vi "VALEW_ATC_Verify Non-concurrent.vi"(0 "GEA2 Reference In":refnum<k24>, 11 "Error In":errorcluster) -> (4 "GEA2 Reference Out":refnum<k24>, 6 "Pass/fail?":bool, 8 "Report Text":string, 15 "Error Out":errorcluster)   [LabVIEW 2016, in "TL27.lvlib"]
doc: "This test covers the ATC algorithm when doing a non-concurrent fill. A non-concurrent fill does not allow both hot and cold valves to be on at the same time. The valves are operated in series, not in parallel."
uses:
  Projects/TL27.lvlib
  C:/Automation/DLLs/PC Dot Net/GeaCommunication.dll
  Common/LabVIEW GEA2 Toolkit/LabVIEW_GEA2_Toolkit.lvlibp/type defs/Source_Destination.ctl
  Valew Common/type defs/MC_Cycle_Engine_Request_State.ctl
  Common/LabVIEW GEA2 Toolkit/LabVIEW_GEA2_Toolkit.lvlibp/type defs/ERD Write Data In.ctl
  Common/LabVIEW GEA2 Toolkit/LabVIEW_GEA2_Toolkit.lvlibp/type defs/Data Type.ctl
  Common/LabVIEW GEA2 Toolkit/LabVIEW_GEA2_Toolkit.lvlibp/type defs/ERD Read Data In.ctl
  <vilib>/DAQmx/write.llb/DAQmx Write (Analog DBL 1Chan 1Samp).vi
  <vilib>/DAQmx/create/channels.llb/DAQmx Create Channel (AO-Voltage-Basic).vi
  <vilib>/DAQmx/miscellaneous.llb/DAQmx Fill In Error Info.vi
  Common/LabVIEW GEA2 Toolkit/LabVIEW_GEA2_Toolkit.lvlibp
panel:
  out "Hot valve time (s) ATC 2":u16
  out "Cold valve time (s) ATC 2":u16
  out "Cold valve time (s) Calc 2":dbl
  out "Hot valve time (s) Calc 2":dbl
  out "High Times (s)":dbl[][](array[numeric])=[[0.048, 19.932000000000002, 0.0], [0.256, 9.626, 10.098], [0.254, 9.628, 10.098], [0.256, 9.625, 10.099], [0.047, 19.933, 0.0], [0.253, 10.701, 9.026], [0.255, 10.699, 9.026], [0.048, 19.932000000000002, 0.0], [0.258, 8.014, 11.708], [0.256, 8.016, 11.708], [0.256, 8.016, 11.708], [0.048, 19.932000000000002, 0.0], [0.254, 7.527, 12.199], [0.047, 19.933, 0.0], [0.253, 6.848, 12.879]]
  out "Hot inlet temp updated after 30sec?":bool
  out "Calc bath temp after seg gals":dbl
  out "Bath temp after seg gals":dbl
  out "Hot valve time (s) ATC":u16
  out "Cold valve time (s) ATC":u16
  out "Bath temp updated after segment fill?":bool
  out "Cold inlet temp updated after 30sec?":bool
  out "Cold valve pass?":bool
  out "Hot valve pass?":bool
  out "Cold valve time (s) Calc":dbl
  out "Hot valve time (s) Calc":dbl
  in  "Standalone?":bool
  # "Segment 1"
  # "Segment 2"
  # "off"
  # "on"
  # "off"
  # "on"
  # "off"
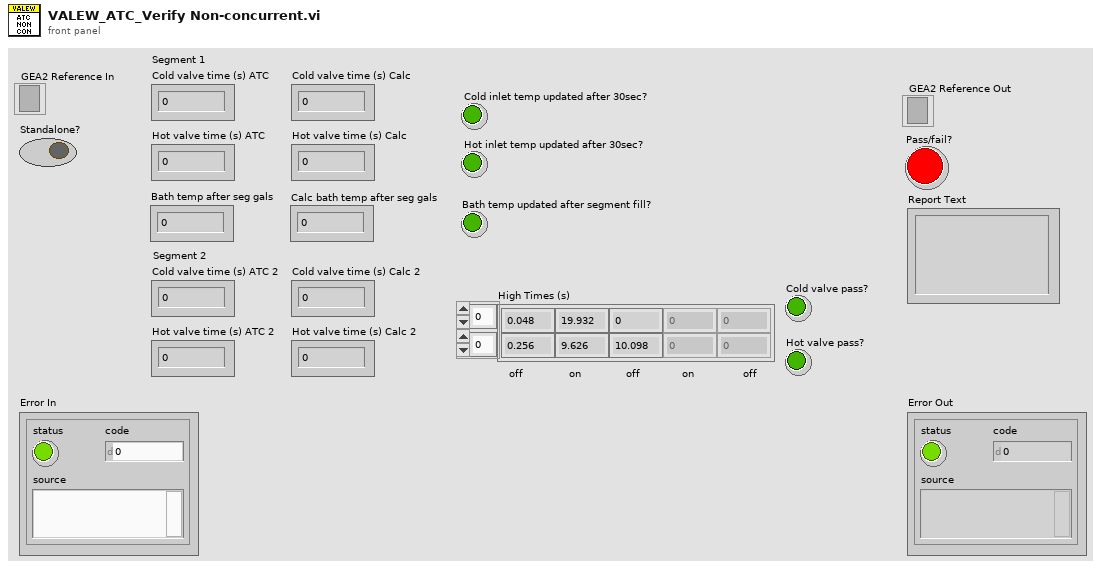
[diagram p1: front panel]
types:
  T1 = typedef "LabVIEW_GEA2_Toolkit.lvlibp/ERD Write Data In.ctl" = cluster{"ERD Number":u16, "Data Type":T2, "Data":string}
  T2 = typedef "LabVIEW_GEA2_Toolkit.lvlibp/Data Type.ctl" = enum16{"string", "boolean", "uint8_t", "uint16_t", "uint32_t", "uint64_t", "int8_t", "int16_t", "int32_t", "int64_t"}
  T3 = typedef "LabVIEW_GEA2_Toolkit.lvlibp/ERD Read Data In.ctl" = cluster{"ERD Number":u16, "Data Type":T2}
  T4 = enum16{"EQ (==)", "NE (!=)", "GT (>)", "LT (<)", "GE (>=)", "LE (<=)", "GTLT(> <)", "GELE (>= <=)", "GELT (>= <)", "GTLE (> <=)", "LTGT (< >)", "LEGE (<= >=)", "LEGT (<= >)", "LTGE (< >=)", "No Comparison"}
  T5 = typedef "TL27.lvlib/MC_Cycle_Engine_Request_State.ctl" = enum16{"Select", "Start", "Pause", "Resume", "Stop"}
  T6 = typedef "LabVIEW_GEA2_Toolkit.lvlibp/Source_Destination.ctl" = cluster{"Source":u8, "Destination":u8}
  T7 = typedef "TL27.lvlib/VALEW_ATC_Data.ctl" = cluster{"Accumulated hot gallons":dbl, "Accumulated cold gallons":dbl, "Current tub gallons":dbl, "Cold inlet temp (F)":dbl, "Hot inlet temp (F)":dbl, "Warm inlet temp (F)":dbl, "Hot valve time (s)":u16, "Cold valve time (s)":u16, "Current bath temp (F)":dbl, "Current water temp (F)":dbl, "Segment gallons":dbl}
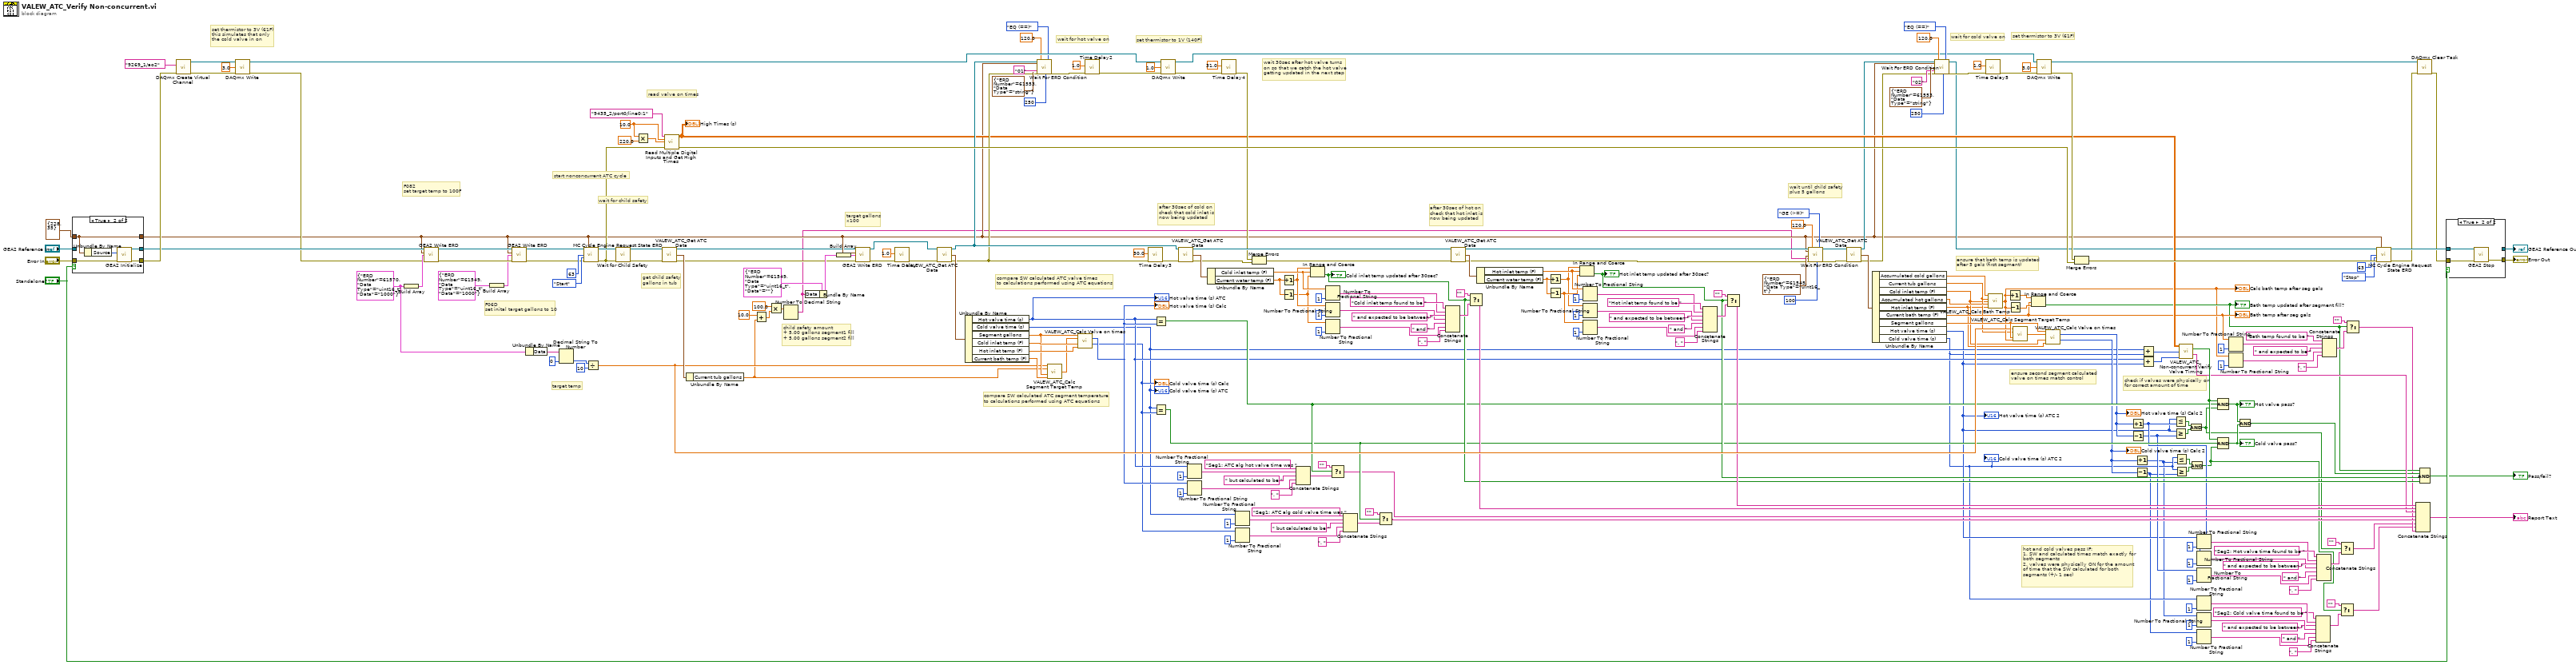
[diagram p0: block diagram]
diagram:
  w199 = 10.0 ("rate")
  w236 = T1 {"ERD Number"=61570, "Data Type"=enum."uint16_t", "Data"="1000"} ("ERD Write Data In")
  # "wait until child safety\nplus 5 gallons"
  # "hot and cold valves pass IF:\n1. SW and calculated times match exactly for\nboth segments\n2. valves were physically ON for the amount\nof time that the SW calculated for both\nsegments (+/- 1 sec)"
  # "compare SW calculated ATC valve times\nto calculations performed using ATC equations"
  # "compare SW calculated ATC segment temperature\nto calculations performed using ATC equations"
  # "wait 30sec after hot valve turns\non so that we catch the hot valve\ngetting updated in the next step"
  # "F06D\nset inital target gallons to 10"
  # "target gallons\nx100"
  # "check if valves were physically on\nfor correct amount of time"
  # "ensure second segment calculated\nvalve on times match control"
  # "ensure that bath temp is updated\nafter 5 gals (first segment)"
  # "wait for cold valve on"
  # "set thermistor to 3V (61F)"
  # "wait for hot valve on"
  # "set thermistor to 1V (140F)"
  # "after 30sec of hot on\ncheck that hot inlet is\nnow being updated"
  # "child safety amount\n+ 5.00 gallons segment1 fill\n+ 5.00 gallons segment2 fill"
  # "after 30sec of cold on\ncheck that cold inlet is\nnow being updated"
  # "get child safety\ngallons in tub"
  # "read valve on times"
  # "target temp"
  # "set thermistor to 3V (61F)\nthis simulates that only\nthe cold valve in on"
  # "wait for child safety"
  # "start nonconcurrent ATC cycle"
  # "F082\nset target temp to 100F"
  n1 = case shown="True" "Standalone?" {
    tunnel: T6 {"Source"=228, "Destination"=35} ("GEA Inputs") -> [w247 w250]
    tunnel: [w249 w253] -> w149
    tunnel: [w248 w252] -> w211
    tunnel: "Error In" -> [w248 w251]
    tunnel: "GEA2 Reference In" -> [w249 _]
    tunnel: [w247 w250] -> w7
    frame False {
    }
    frame True {
      n2 = Unbundle By Name(w250) -> ("Source"=w254:u8)
      n3 = call "GEA2 Initialize.vi"("Source Address"=w254, "error in"=w251) -> ("GEA2 Reference Out"=w253:refnum<k24>, "error out"=w252:errorcluster)  [unwired: 11 in, 1 out]
    }
  }
  n4 = call-poly <vilib>:"DAQmx Create Virtual Channel.vi"("physical channels"=tag "9269_1/ao2", "error in"=w211) -> ("task out"=w228:refnum<k21>, "error out"=w227:errorcluster)  [unwired: 12 in]
  n5 = call-poly <vilib>:"DAQmx Write.vi"("task/channels in"=w228, "data"=3.0, "error in"=w227) -> ("task out"=w196:refnum<k21>, "error out"=w148:errorcluster)  [unwired: 10 in, 1 out]
  n6 = Build Array(w236) -> (w235:T1[])
  n7 = call "GEA2 Write ERD.vi"("GEA2 Reference In"=w149, "GEA Inputs"=w7, "Write ERD List"=w235, "Error In"=w148) -> ("GEA2 Reference Out"=w224:refnum<k24>, "Error Out"=w223:errorcluster)  [unwired: 9 in, 1 out]
  n8 = Build Array(T1 {"ERD Number"=61549, "Data Type"=enum."uint16_t", "Data"="1000"} ("ERD Write Data In")) -> (w207:T1[])
  n9 = call "GEA2 Write ERD.vi"("GEA2 Reference In"=w224, "GEA Inputs"=w7, "Write ERD List"=w207, "Error In"=w223) -> ("GEA2 Reference Out"=w221:refnum<k24>, "Error Out"=w222:errorcluster)  [unwired: 9 in, 1 out]
  n10 = Unbundle By Name(w236) -> ("Data"=w234:string)
  n11 = Decimal String To Number(string=w234, default (0L)=u16 0 ("default (0 U32)")) -> (number=w232:u16)  [unwired: 1 in, 1 out]
  n12 = call "MC Cycle Engine Request State ERD.vi"("GEA2 Reference In"=w221, "GEA Inputs"=w7, "Cycle #"=u8 63, "MC Cycle Engine State"=MC_Cycle_Engine_Request_State."Start", "Error In"=w222) -> ("GEA2 Reference Out"=w241:refnum<k24>, "Error Out"=w160:errorcluster)  [unwired: 9 in]
  n13 = Divide(x=w232, y=u16 10) -> (x/y=w154:dbl)
  n14 = call "Wait for Child Safety.vi"("GEA2 Reference In"=w241, "Error In"=w160) -> ("GEA2 Reference Out"=w220:refnum<k24>, "Error Out"=w195:errorcluster)  [unwired: 9 in, 3 out]
  n15 = Multiply(x=w199, y=220.0) -> (x*y=w200:dbl)
  n16 = call "VALEW_ATC_Get ATC Data.vi"("GEA2 Reference In"=w220, "Error In"=w195) -> ("GEA2 Reference Out"=w2:refnum<k24>, "ATC Data"=w219:T7, "Error Out"=w5:errorcluster)  [unwired: 11 in]
  n17 = call "Read Multiple Digital Inputs and Get High Times.vi"("Lines"=tag "9435_2/port0/line0:1", "Rate (Hz)"=w199, "Samples"=w200, "Error In"=w160) -> ("High Times (s)"=w159:dbl[][], "Error Out"=w198:errorcluster)  [unwired: 10 in]
  "High Times (s)" <- w159
  n18 = Unbundle By Name(w219) -> ("Current tub gallons"=w6:dbl)
  n19 = Add(x=10.0, y=w6) -> (x+y=w9:dbl)
  n20 = Multiply(x=100.0, y=w9) -> (x*y=w10:dbl)
  n21 = Number To Decimal String(number=w10) -> (decimal integer string=w1:string)  [unwired: 1 in]
  n22 = Bundle By Name(cluster=T1 {"ERD Number"=61549, "Data Type"=enum."uint16_t", "Data"=""} ("ERD Write Data In"), "Data"=w1) -> (w11:T1)
  n23 = Build Array(w11) -> (w14:T1[])
  n24 = call "GEA2 Write ERD.vi"("GEA2 Reference In"=w2, "GEA Inputs"=w7, "Write ERD List"=w14, "Error In"=w5) -> ("GEA2 Reference Out"=w3:refnum<k24>, "Error Out"=w4:errorcluster)  [unwired: 9 in, 1 out]
  n25 = call "Time Delay"("error in (no error)"=w4, "Delay Time (s)"=1.0) -> ("error out"=w239:errorcluster)  [unwired: 9 in]
  n26 = call "VALEW_ATC_Get ATC Data.vi"("GEA2 Reference In"=w3, "Error In"=w239) -> ("GEA2 Reference Out"=w178:refnum<k24>, "ATC Data"=w238:T7, "Error Out"=w170:errorcluster)  [unwired: 11 in]
  n27 = Unbundle By Name(w238) -> ("Hot valve time (s)"=w29:u16, "Cold valve time (s)"=w27:u16, "Segment gallons"=w209:dbl, "Cold inlet temp (F)"=w217:dbl, "Hot inlet temp (F)"=w237:dbl, "Current bath temp (F)"=w208:dbl)
  "Cold valve time (s) ATC" <- w27
  "Hot valve time (s) ATC" <- w29
  n28 = call "Wait For ERD Condition.vi"("GEA2 Reference In"=w178, "GEA Inputs"=w7, "ERD Read Data"=T3 {"ERD Number"=61553, "Data Type"=enum."string"}, "Expected Low"="01", "Error In"=w170, "Timeout (s)"=120.0, "Loop Rate (ms)"=u32 250, "Comparison"=T4."EQ (==)") -> ("Error Out"=w167:errorcluster)  [unwired: 7 in, 4 out]
  n29 = call "VALEW_ATC_Calc Segment Target Temp.vi"("T(target)"=w154, "V(bath)"=w6, "V(segment)"=w209, "T(bath)"=w208) -> ("T(segment target)"=w210:dbl)  [unwired: 11 in]
  n30 = call "VALEW_ATC_Calc Valve on times.vi"("V(segment)"=w209, "T(segment target)"=w210, "T(cold inlet)"=w217, "T(hot inlet)"=w237) -> ("t(hot valve)"=w30:u16, "t(cold valve)"=w28:u16)  [unwired: 10 in]
  "Hot valve time (s) Calc" <- w30
  "Cold valve time (s) Calc" <- w28
  n31 = call "Time Delay2"("error in (no error)"=w167, "Delay Time (s)"=1.0) -> ("error out"=w168:errorcluster)  [unwired: 9 in]
  n32 = call "Time Delay3"("error in (no error)"=w170, "Delay Time (s)"=30.0) -> ("error out"=w193:errorcluster)  [unwired: 9 in]
  n33 = Equal?(x=w29, y=w30) -> (x = y?=w75:bool)
  n34 = Equal?(x=w27, y=w28) -> (x = y?=w74:bool)
  n35 = call-poly <vilib>:"DAQmx Write.vi"("task/channels in"=w196, "data"=1.0, "error in"=w168) -> ("task out"=w171:refnum<k21>, "error out"=w191:errorcluster)  [unwired: 10 in, 1 out]
  n36 = call "VALEW_ATC_Get ATC Data.vi"("GEA2 Reference In"=w178, "Error In"=w193) -> ("GEA2 Reference Out"=w188:refnum<k24>, "ATC Data"=w229:T7, "Error Out"=w185:errorcluster)  [unwired: 11 in]
  n37 = Number To Fractional String(number=w29, precision (6)=i16 1) -> (F-format string=w91:string)  [unwired: 2 in]
  n38 = Number To Fractional String(number=w30, precision (6)=i16 1) -> (F-format string=w89:string)  [unwired: 2 in]
  n39 = Unbundle By Name(w229) -> ("Cold inlet temp (F)"=w110:dbl, "Current water temp (F)"=w216:dbl)
  n40 = call "Time Delay4"("error in (no error)"=w191, "Delay Time (s)"=31.0) -> ("error out"=w163:errorcluster)  [unwired: 9 in]
  n41 = Number To Fractional String(number=w27, precision (6)=i16 1) -> (F-format string=w78:string)  [unwired: 2 in]
  n42 = Number To Fractional String(number=w28, precision (6)=i16 1) -> (F-format string=w80:string)  [unwired: 2 in]
  n43 = Merge Errors(w163, w185) -> (w186:errorcluster)
  n44 = Increment(x=w216) -> (x+1=w109:dbl)
  n45 = Decrement(x=w216) -> (x-1=w108:dbl)
  n46 = Concatenate Strings("Seg1: ATC alg hot valve time was ", w91, " but calculated to be ", w89, ". " ("string")) -> (w86:string)
  n47 = In Range and Coerce(upper limit=w109, x=w110, lower limit=w108) -> (In Range?=w95:bool)  [unwired: 1 out]
  "Cold inlet temp updated after 30sec?" <- w95
  n48 = Number To Fractional String(number=w110, precision (6)=i16 1) -> (F-format string=w114:string)  [unwired: 2 in]
  n49 = Number To Fractional String(number=w109, precision (6)=i16 1) -> (F-format string=w113:string)  [unwired: 2 in]
  n50 = Number To Fractional String(number=w108, precision (6)=i16 1) -> (F-format string=w132:string)  [unwired: 2 in]
  n51 = Select(t="", s=w75, f=w86) -> (s? t:f=w72:string)
  n52 = Concatenate Strings("Seg1: ATC alg cold valve time was ", w78, " but calculated to be ", w80, ". " ("string")) -> (w83:string)
  n53 = Select(t="", s=w74, f=w83) -> (s? t:f=w73:string)
  n54 = Concatenate Strings("Cold inlet temp found to be ", w114, " and expected to be between ", w113, " and " ("string"), w132, ". " ("string")) -> (w134:string)
  n55 = call "VALEW_ATC_Get ATC Data.vi"("GEA2 Reference In"=w188, "Error In"=w186) -> ("GEA2 Reference Out"=w60:refnum<k24>, "ATC Data"=w189:T7, "Error Out"=w59:errorcluster)  [unwired: 11 in]
  n56 = Select(t="", s=w95, f=w134) -> (s? t:f=w104:string)
  n57 = Unbundle By Name(w189) -> ("Hot inlet temp (F)"=w107:dbl, "Current water temp (F)"=w190:dbl)
  n58 = Increment(x=w190) -> (x+1=w105:dbl)
  n59 = Decrement(x=w190) -> (x-1=w106:dbl)
  n60 = In Range and Coerce(upper limit=w105, x=w107, lower limit=w106) -> (In Range?=w96:bool)  [unwired: 1 out]
  "Hot inlet temp updated after 30sec?" <- w96
  n61 = Number To Fractional String(number=w107, precision (6)=i16 1) -> (F-format string=w112:string)  [unwired: 2 in]
  n62 = Number To Fractional String(number=w105, precision (6)=i16 1) -> (F-format string=w111:string)  [unwired: 2 in]
  n63 = Number To Fractional String(number=w106, precision (6)=i16 1) -> (F-format string=w117:string)  [unwired: 2 in]
  n64 = Concatenate Strings("Hot inlet temp found to be ", w112, " and expected to be between ", w111, " and " ("string"), w117, ". " ("string")) -> (w115:string)
  n65 = Select(t="", s=w96, f=w115) -> (s? t:f=w103:string)
  n66 = call "Wait For ERD Condition.vi"("GEA2 Reference In"=w60, "GEA Inputs"=w7, "ERD Read Data"=T3 {"ERD Number"=61545, "Data Type"=enum."uint16_t"}, "Expected Low"=w1, "Error In"=w59, "Timeout (s)"=120.0, "Loop Rate (ms)"=u32 100, "Comparison"=T4."GE (>=)") -> ("GEA2 Reference Out"=w66:refnum<k24>, "Error Out"=w65:errorcluster)  [unwired: 7 in, 3 out]
  n67 = call "VALEW_ATC_Get ATC Data.vi"("GEA2 Reference In"=w66, "Error In"=w65) -> ("GEA2 Reference Out"=w153:refnum<k24>, "ATC Data"=w218:T7, "Error Out"=w151:errorcluster)  [unwired: 11 in]
  n68 = Unbundle By Name(w218) -> ("Accumulated cold gallons"=w214:dbl, "Current tub gallons"=w63:dbl, "Cold inlet temp (F)"=w62:dbl, "Accumulated hot gallons"=w215:dbl, "Hot inlet temp (F)"=w61:dbl, "Current bath temp (F)"=w135:dbl, "Segment gallons"=w155:dbl, "Hot valve time (s)"=w22:u16, "Cold valve time (s)"=w17:u16)
  "Bath temp after seg gals" <- w135
  "Cold valve time (s) ATC 2" <- w17
  "Hot valve time (s) ATC 2" <- w22
  n69 = call "Wait For ERD Condition.vi"("GEA2 Reference In"=w153, "GEA Inputs"=w7, "ERD Read Data"=T3 {"ERD Number"=61553, "Data Type"=enum."string"}, "Expected Low"="02", "Error In"=w151, "Timeout (s)"=120.0, "Loop Rate (ms)"=u32 250, "Comparison"=T4."EQ (==)") -> ("GEA2 Reference Out"=w152:refnum<k24>, "Error Out"=w165:errorcluster)  [unwired: 7 in, 3 out]
  n70 = call "Time Delay5"("error in (no error)"=w165, "Delay Time (s)"=1.0) -> ("error out"=w164:errorcluster)  [unwired: 9 in]
  n71 = call "VALEW_ATC_Calc Bath Temp.vi"("V(bath cold)"=w214, "V(bath)"=w63, "T(cold inlet)"=w62, "V(bath hot)"=w215, "T(hot inlet)"=w61) -> ("T(bath)"=w64:dbl)  [unwired: 10 in]
  "Calc bath temp after seg gals" <- w64
  n72 = Increment(x=w64) -> (x+1=w212:dbl)
  n73 = Decrement(x=w64) -> (x-1=w213:dbl)
  n74 = call "VALEW_ATC_Calc Segment Target Temp.vi"("T(target)"=w154, "V(bath)"=w63, "V(segment)"=w155, "T(bath)"=w64) -> ("T(segment target)"=w156:dbl)  [unwired: 11 in]
  n75 = In Range and Coerce(upper limit=w212, x=w135, lower limit=w213) -> (In Range?=w100:bool)  [unwired: 1 out]
  "Bath temp updated after segment fill?" <- w100
  n76 = call-poly <vilib>:"DAQmx Write.vi"("task/channels in"=w171, "data"=3.0, "error in"=w164) -> ("task out"=w162:refnum<k21>, "error out"=w161:errorcluster)  [unwired: 10 in, 1 out]
  n77 = call "VALEW_ATC_Calc Valve on times.vi"("V(segment)"=w155, "T(segment target)"=w156, "T(cold inlet)"=w62, "T(hot inlet)"=w61) -> ("t(hot valve)"=w46:u16, "t(cold valve)"=w44:u16)  [unwired: 10 in]
  "Hot valve time (s) Calc 2" <- w46
  "Cold valve time (s) Calc 2" <- w44
  n78 = Merge Errors(w161, w198) -> (w202:errorcluster)
  n79 = Increment(x=w46) -> (x+1=w24:u16)
  n80 = Decrement(x=w46) -> (x-1=w23:u16)
  n81 = Increment(x=w44) -> (x+1=w16:u16)
  n82 = Decrement(x=w44) -> (x-1=w15:u16)
  n83 = Add(x=w27, y=w17) -> (x+y=w158:u16)
  n84 = Add(x=w29, y=w22) -> (x+y=w157:u16)
  n85 = Less Or Equal?(x=w22, y=w24) -> (x <= y?=w26:bool)
  n86 = Greater Or Equal?(x=w22, y=w23) -> (x >= y?=w25:bool)
  n87 = Less Or Equal?(x=w17, y=w16) -> (x <= y?=w19:bool)
  n88 = Greater Or Equal?(x=w17, y=w15) -> (x >= y?=w20:bool)
  n89 = call "VALEW_ATC_Non-concurrent Verify Valve Timing.vi"("High Times (s)"=w159, "Total cold ON time (s)"=w158, "Total hot ON time (s)"=w157) -> ("Pass/Fail?"=w150:bool, "Report Text"=w102:string)  [unwired: 11 in]
  n90 = And(x=w26, y=w25) -> (x .and. y?=w21:bool)
  n91 = And(x=w19, y=w20) -> (x .and. y?=w18:bool)
  n92 = Number To Fractional String(number=w17, precision (6)=i16 1) -> (F-format string=w42:string)  [unwired: 2 in]
  n93 = Number To Fractional String(number=w16, precision (6)=i16 1) -> (F-format string=w43:string)  [unwired: 2 in]
  n94 = Number To Fractional String(number=w15, precision (6)=i16 1) -> (F-format string=w34:string)  [unwired: 2 in]
  n95 = Number To Fractional String(number=w22, precision (6)=i16 1) -> (F-format string=w48:string)  [unwired: 2 in]
  n96 = Number To Fractional String(number=w24, precision (6)=i16 1) -> (F-format string=w47:string)  [unwired: 2 in]
  n97 = Number To Fractional String(number=w23, precision (6)=i16 1) -> (F-format string=w56:string)  [unwired: 2 in]
  n98 = Compound Arithmetic op=AND(w150, w75, w21) -> (w99:bool)
  "Hot valve pass?" <- w99
  n99 = Compound Arithmetic op=AND(w150, w74, w18) -> (w98:bool)
  "Cold valve pass?" <- w98
  n100 = Number To Fractional String(number=w135, precision (6)=i16 1) -> (F-format string=w140:string)  [unwired: 2 in]
  n101 = Number To Fractional String(number=w64, precision (6)=i16 1) -> (F-format string=w138:string)  [unwired: 2 in]
  n102 = And(x=w99, y=w98) -> (x .and. y?=w97:bool)
  n103 = Concatenate Strings("Seg2: Cold valve time found to be ", w42, " and expected to be between ", w43, " and " ("string"), w34, ". " ("string")) -> (w32:string)
  n104 = Concatenate Strings("Seg2: Hot valve time found to be ", w48, " and expected to be between ", w47, " and " ("string"), w56, ". " ("string")) -> (w58:string)
  n105 = Concatenate Strings("Bath temp found to be ", w140, " and expected to be ", w138, ". " ("string")) -> (w137:string)
  n106 = Select(t="", s=w18, f=w32) -> (s? t:f=w31:string)
  n107 = Select(t="", s=w21, f=w58) -> (s? t:f=w45:string)
  n108 = Select(t="", s=w100, f=w137) -> (s? t:f=w71:string)
  n109 = call "MC Cycle Engine Request State ERD.vi"("GEA2 Reference In"=w152, "GEA Inputs"=w7, "Cycle #"=u8 63, "MC Cycle Engine State"=MC_Cycle_Engine_Request_State."Stop", "Error In"=w202) -> ("GEA2 Reference Out"=w201:refnum<k24>, "Error Out"=w187:errorcluster)  [unwired: 9 in]
  n110 = Concatenate Strings(w103, w104, w102, w72, w73, w45, w31, w71) -> (→"Report Text":string)
  n111 = call <vilib>:"DAQmx Clear Task.vi"("task in"=w162, "error in"=w187) -> ("error out"=w145:errorcluster)  [unwired: 13 in]
  n112 = Compound Arithmetic op=AND(w100, w97, w96, w95) -> (→"Pass/fail?":bool)
  n113 = case shown="True" "Standalone?" {
    tunnel: w145 -> [w256 w259]
    tunnel: w201 -> [w255 w258]
    tunnel: [w256 w257] -> w204
    tunnel: [w255 _] -> w205
    frame False {
    }
    frame True {
      n114 = call "GEA2 Stop.vi"("GEA2 Reference In"=w258, "Error In"=w259) -> ("Error Out"=w257:errorcluster)  [unwired: 13 in]
    }
  }
  "GEA2 Reference Out" <- w205
  "Error Out" <- w204
